vi "IsArmed.vi"(8 "error in (no error)":errorcluster, 11 "NI-Scope Digitizer in":refnum<class "Ni-Scope Digitizer.lvclass">) -> (0 "error out":errorcluster, 1 "Finished":bool, 2 "Armed":bool, 3 "NI-Scope Digitizer out":refnum<class "Ni-Scope Digitizer.lvclass">, 4 "Availiable Samples":u32)   [LabVIEW 2015, in "Ni-Scope Digitizer.lvclass"]
uses:
  Ni-Scope Digitizer.lvclass
  Ni-Scope Digitizer.lvclass/Ni-Scope Digitizer.ctl
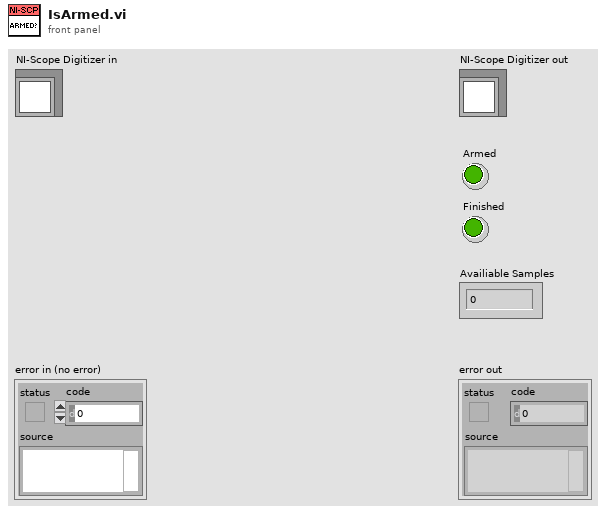
[diagram p1: front panel]
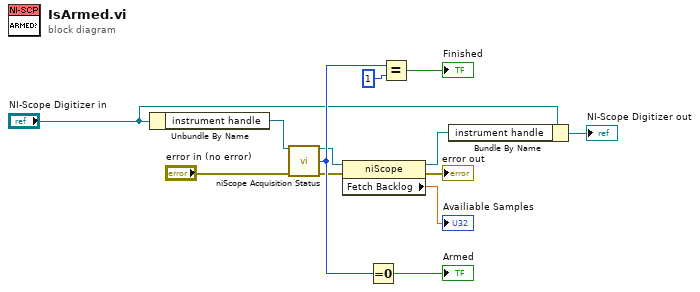
[diagram p0: block diagram]
diagram:
  n1 = Unbundle By Name("NI-Scope Digitizer in") -> ("instrument handle"=w13:refnum<k15>)
  n2 = call <instrlib>:"niScope Acquisition Status.vi"("instrument handle"=w13, "error in"="error in (no error)") -> ("instrument handle out"=w6:refnum<k15>, "acquisition status"=w10:i32, "error out"=w5:errorcluster)  [unwired: 11 out]
  n3 = property class="niScope"(reference=w6, error in=w5) -> (reference out=w2:refnum<k15>, error out=→"error out":errorcluster, "Fetch Backlog"=→"Availiable Samples":dbl)
  n4 = Equal To 0?(x=w10) -> (x = 0?=→"Armed":bool)
  n5 = Equal?(x=w10, y=1) -> (x = y?=→"Finished":bool)
  n6 = Bundle By Name(cluster="NI-Scope Digitizer in", "instrument handle"=w2) -> (→"NI-Scope Digitizer out":refnum<class "Ni-Scope Digitizer.lvclass">)
